vi "roboRIO v1.0 Reserve AI.vi"(7 "Allow multiple opens?":bool, 8 "error in (no error)":errorcluster, 10 "AI Channel List":T1) -> (0 "error out":errorcluster)   [LabVIEW 2021]
uses:
  <vilib>/myRIO/Common/Instrument Driver Framework/myRIO v1.0/AI/typedefs/AI Channels List.ctl
  <vilib>/myRIO/Common/Instrument Driver Framework/myRIO v1.0/AI/typedefs/AI Channels Enum.ctl
  <vilib>/myRIO/Common/Instrument Driver Framework/roboRIO v1.0/Resource Manager/vis/roboRIO v1.0 Reserve Channel.vi
  <vilib>/myRIO/Common/Instrument Driver Framework/roboRIO v1.0/Resource Manager/vis/roboRIO v1.0 Unreserve Channel.vi
  <vilib>/myRIO/Common/Instrument Driver Framework/roboRIO v1.0/Resource Manager/vis/roboRIO v1.0 Build Mutex Name.vi
  <vilib>/myRIO/Common/Instrument Driver Framework/Utilities/vis/IO Manager.vi
  <vilib>/Utility/error.llb/Error Cluster From Error Code.vi
  <vilib>/myRIO/Common/Instrument Driver Framework/Utilities/vis/Configuration Manager.vi
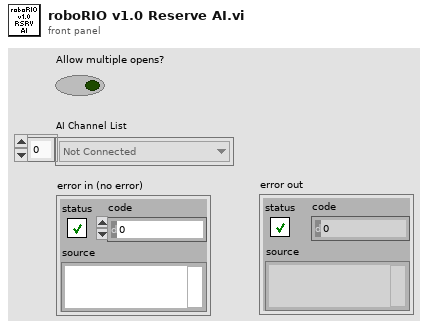
[diagram p1: front panel]
types:
  T1 = typedef "AI Channels List.ctl" = T2[]
  T2 = typedef "AI Channels Enum.ctl" = enum16{"Not Connected", "AudioIn/Left", "AudioIn/Right", "C/AI0", "C/AI1", "A/AI0", "A/AI1", "A/AI2", "A/AI3", "A/AI4", "A/AI5", "A/AI6", "A/AI7", "B/AI0", "B/AI1", "B/AI2", "B/AI3", "B/AI4", "B/AI5", "B/AI6", "B/AI7", "AI/AI0", "AI/AI1", "AI/AI2", "AI/AI3", "A/AI0 (DIFF)", "A/AI1 (DIFF)", "A/AI2 (DIFF)", "A/AI3 (DIFF)", "B/AI0 (DIFF)", "B/AI1 (DIFF)", "B/AI2 (DIFF)", "B/AI3 (DIFF)"}
  T3 = typedef "roboRIO v1.0 Channel Reservation List.ctl" = T4[]
  T4 = typedef "roboRIO v1.0 Channel Reservation Info.ctl" = cluster{"Channel Name":string, "Connector":T5, "Mutex ID":i32}
  T5 = typedef "roboRIO v1.0 Connector List.ctl" = enum32{"None", "ConnectorB", "ConnectorI2C", "ConnectorDIO", "ConnectorRSL", "ConnectorRELAY", "ConnectorAI", "ConnectorPWM", "ConnectorSPI"}
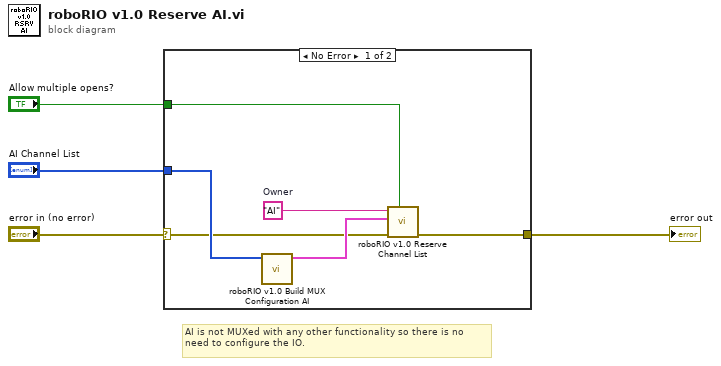
[diagram p0: block diagram]
diagram:
  # "AI is not MUXed with any other functionality so there is no need to configure the IO."
  n1 = case shown="No Error" "error in (no error)" {
    selector: "error in (no error)" -> [w7 w11]
    tunnel: "Allow multiple opens?" -> [w6 _]
    tunnel: "AI Channel List" -> [w10 _]
    tunnel: [w5 w11] -> w3
    frame No Error {
      w9 = "AI"  # Owner
      n2 = call <vilib>:"roboRIO v1.0 Build MUX Configuration AI.vi"("AI Channels List"=w10) -> ("Channel Reservation Info"=w8:T3)  [unwired: 10 in]
      n3 = call <vilib>:"roboRIO v1.0 Reserve Channel List.vi"("Allow multiple opens?"=w6, "error in (no error)"=w7, "Channel Reservation List"=w8, "Owner"=w9) -> ("error out"=w5:errorcluster)  [unwired: 7 in]
    }
    frame Error {
      # "There is an incoming error so there is nothing to do."
    }
  }
  "error out" <- w3
